vi "3_termometro_DAQ.vi"() -> ()   [LabVIEW 2017]
panel:
  out "ITERA钦ES":i32
  in  "stop":bool
  out "Kelvin":dbl(slide) scale=0.0..350.0
  out "Fahrenheit":dbl(slide) scale=0.0..150.0
  # "CONVERSÃO DE ESCALAS TERMOMÉTRICAS"
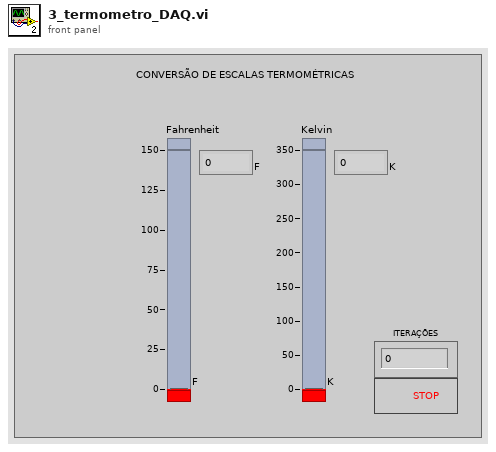
[diagram p1: front panel]
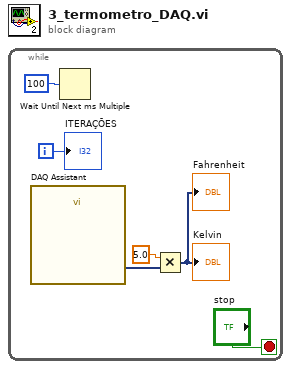
[diagram p0: block diagram]
diagram:
  n1 = while {
    i -> [w3]
    stop <- "stop" stop-if-true
    n2 = call "DAQ Assistant"() -> ("data"=w5:dynamicdata)  [unwired: 17 in, 2 out]
    n3 = Wait Until Next ms Multiple(millisecond multiple=u32 100) -> ()  [unwired: 1 out]
    n4 = Multiply(x=5.0, y=w5) -> (x*y=→"Fahrenheit" →"Kelvin":dynamicdata)
    "ITERA钦ES" <- w3
  }
